vi "_Read with Timeout.vi"(8 "error in (no error)":errorcluster, 9 "timeout (ms) out":i32, 11 "read fd":u64 format="%016x") -> (0 "error out 2":errorcluster, 1 "read eof?":bool, 2 "read data":u8[](array[numeric]), 3 "read fd out":u64 format="%016x")   [LabVIEW 2020, in "NI_Subprocess.lvlib" / "Subprocess.lvclass"]
uses:
  <vilib>/Subprocess/Subprocess/Subprocess.lvclass
  lviosrg.dll
  <vilib>/ErrorRing/Error Ring.xnode
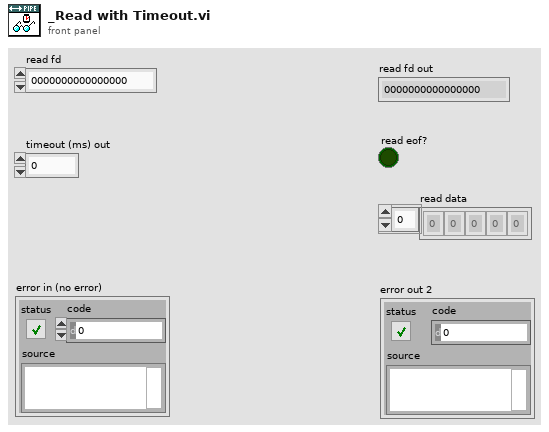
[diagram p1: front panel]
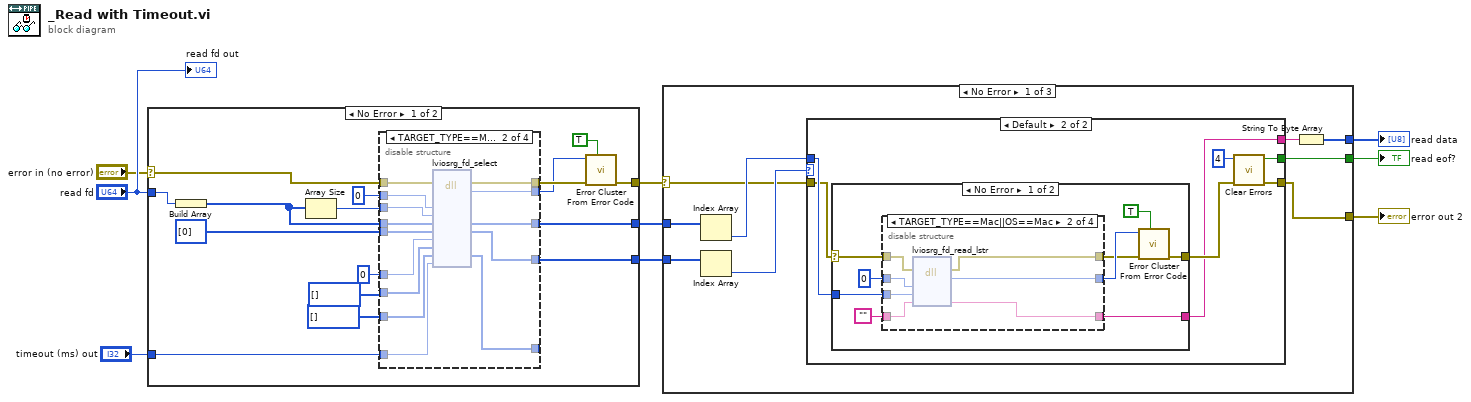
[diagram p0: block diagram]
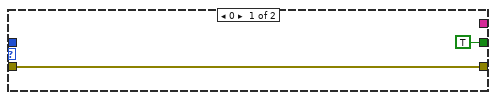
[diagram p2: hidden frame]
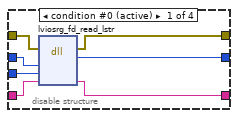
[diagram p3: hidden frame]
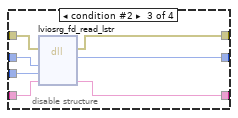
[diagram p4: hidden frame]
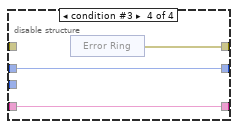
[diagram p5: hidden frame]
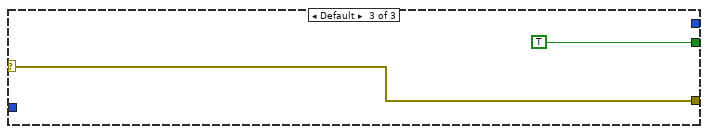
[diagram p8: hidden frame]
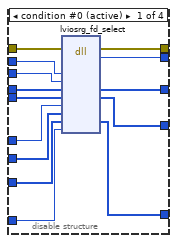
[diagram p9: hidden frame]
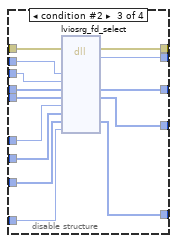
[diagram p10: hidden frame]
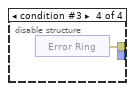
[diagram p11: hidden frame]
diagram:
  n1 = case shown="No Error" "error in (no error)" {
    selector: "error in (no error)" -> [w20 w73]
    tunnel: "read fd" -> [w19 _]
    tunnel: [w23 _] -> w4
    tunnel: [w17 w73] -> w2
    tunnel: [w22 _] -> w3
    tunnel: "timeout (ms) out" -> [w10 _]
    frame No Error {
      n2 = Build Array(w19) -> (w12:u64[])
      n3 = Array Size(array=w12) -> (size(s)=w24:i32)
      n4 = disable-structure "Conditional Disable Structure" shown="TARGET_TYPE==Mac||OS==Mac" {
        disable-tunnel: 0 ("errno") -> [w39 w53 w67 _]
        disable-tunnel: w12 -> [w38 w52 w57 _]
        disable-tunnel: w24 -> [w37 w51 w66 _]
        disable-tunnel: 0 -> [w36 w50 w65 _]
        disable-tunnel: u64[] [] -> [w30 w42 w59 _]
        disable-tunnel: w10 -> [w35 w49 w64 _]
        disable-tunnel: [w28 w48 w63 _] -> w22
        disable-tunnel: [w29 w47 w62 _] -> w23
        disable-tunnel: [w34 w46 w61 w68] -> w21
        disable-tunnel: w20 -> [w33 w45 w60 _]
        disable-tunnel: [w32 w43 w58 _] -> w18
        disable-tunnel: u8[] [0] ("write_fds") -> [w31 w44 w56 _]
        disable-tunnel: u8[] [] -> [w27 w41 w55 _]
        disable-tunnel: [w26 w40 w54 _] -> _
        frame condition #0 (active) {
          n5 = dll-call lib="lviosrg.*" fn="lviosrg_fd_select"(error in=w33, "errno"=w39, "readCnt"=w37, "read_fds"=w38, "read_fds_ready"=w31, "writeCnt"=w36, "write_fds"=w30, "write_fds_ready"=w27, "timeOut"=w35) -> (error out=w34:errorcluster, "return type"=w32:i32, "read_fds"=w29:u64[], "read_fds_ready"=w28:u8[], "write_fds_ready"=w26:i32[])  [unwired: 9 in, 1 out]
        }
        frame condition #1 {
          n6 = dll-call lib="lviosrg.*" fn="lviosrg_fd_select"(error in=w45, "errno"=w53, "readCnt"=w51, "read_fds"=w52, "read_fds_ready"=w44, "writeCnt"=w50, "write_fds"=w42, "write_fds_ready"=w41, "timeOut"=w49) -> (error out=w46:errorcluster, "return type"=w43:i32, "read_fds"=w47:u64[], "read_fds_ready"=w48:u8[], "write_fds_ready"=w40:i32[])  [unwired: 9 in, 1 out]
        }
        frame condition #2 {
          n7 = dll-call lib="lviosrg.*" fn="lviosrg_fd_select"(error in=w60, "errno"=w67, "readCnt"=w66, "read_fds"=w57, "read_fds_ready"=w56, "writeCnt"=w65, "write_fds"=w59, "write_fds_ready"=w55, "timeOut"=w64) -> (error out=w61:errorcluster, "return type"=w58:i32, "read_fds"=w62:u64[], "read_fds_ready"=w63:u8[], "write_fds_ready"=w54:i32[])  [unwired: 9 in, 1 out]
        }
        frame condition #3 {
          n8 = xnode ("Error Ring")() -> ("error out"=w68:errorcluster)
        }
      }
      n9 = call <vilib>:"Error Cluster From Error Code.vi"("show call chain? (False)"=TRUE, "error in (no error)"=w21, "error code (0)"=w18) -> ("error out"=w17:errorcluster)  [unwired: 6 in]
    }
    frame Error {
    }
  }
  n10 = case shown="No Error" w2 {
    selector: w2 -> [w80 w130 w132]
    tunnel: w4 -> [w75 _ _]
    tunnel: w3 -> [w74 _ _]
    tunnel: [w76 w130 w132] -> w6
    tunnel: [w78 _ _] -> w8
    tunnel: [w77 _ TRUE] -> w7
    frame No Error {
      n11 = Index Array(array=w75) -> (element=w82:u64)  [unwired: 1 in]
      n12 = Index Array(array=w74) -> (element=w81:u8)  [unwired: 1 in]
      n13 = case shown="Default" w81 {
        tunnel: w82 -> [_ w88]
        tunnel: w80 -> [w84 w85]
        tunnel: [w84 w89] -> w76
        tunnel: [_ w86] -> w79
        tunnel: [TRUE ("specific error cleared?") w90] -> w77
        frame 0 {
        }
        frame Default {
          n14 = case shown="No Error" w85 {
            selector: w85 -> [w97 w129]
            tunnel: [w93 w129] -> w87
            tunnel: [w100 _] -> w86
            tunnel: w88 -> [w92 _]
            frame No Error {
              n15 = disable-structure shown="TARGET_TYPE==Mac||OS==Mac" {
                disable-tunnel: [w107 w114 w121 w122] -> w94
                disable-tunnel: w97 -> [w106 w113 w120 _]
                disable-tunnel: [w105 w112 w119 w124] -> w100
                disable-tunnel: w92 -> [w104 w108 w118 _]
                disable-tunnel: "" -> [w103 w111 w117 w124]
                disable-tunnel: [w102 w110 w116 w123] -> w95
                disable-tunnel: 0 ("errno") -> [w101 w109 w115 w123]
                frame condition #0 (active) {
                  n16 = dll-call lib="lviosrg.*" fn="lviosrg_fd_read_lstr"(error in=w106, "errno"=w101, "read_fd"=w104, "buf"=w103) -> (error out=w107:errorcluster, "return type"=w102:i32, "buf"=w105:string)  [unwired: 4 in, 1 out]
                }
                frame condition #1 {
                  n17 = dll-call lib="lviosrg.*" fn="lviosrg_fd_read_lstr"(error in=w113, "errno"=w109, "read_fd"=w108, "buf"=w111) -> (error out=w114:errorcluster, "return type"=w110:i32, "buf"=w112:string)  [unwired: 4 in, 1 out]
                }
                frame condition #2 {
                  n18 = dll-call lib="lviosrg.*" fn="lviosrg_fd_read_lstr"(error in=w120, "errno"=w115, "read_fd"=w118, "buf"=w117) -> (error out=w121:errorcluster, "MgErr"=w116:i32, "buf"=w119:string)  [unwired: 4 in, 1 out]
                }
                frame condition #3 {
                  n19 = xnode "Error Ring"() -> ("error out"=w122:errorcluster)
                }
              }
              n20 = call <vilib>:"Error Cluster From Error Code.vi"("show call chain? (False)"=TRUE, "error in (no error)"=w94, "error code (0)"=w95) -> ("error out"=w93:errorcluster)  [unwired: 6 in]
            }
            frame Error {
            }
          }
          n21 = call <vilib>:"Clear Errors.vi"("error in (no error)"=w87, "specific error code to clear (0: all)"=4) -> ("error out"=w89:errorcluster, "specific error cleared?"=w90:bool)  [unwired: 4 in]
        }
      }
      n22 = String To Byte Array(string=w79) -> (unsigned byte array=w78:u8[])
    }
    frame Error {
    }
    frame Default {
    }
  }
  "error out 2" <- w6
  "read eof?" <- w7
  "read data" <- w8
  "read fd out" <- "read fd"
